vi "Update LCD.vi"(8 "error in":errorcluster, 11 "Data Cluster":T1) -> (0 "error out":errorcluster, 2 "LCD":string, 3 "Module Data":T1)   [LabVIEW 2026, in "Front Panel Emulator.lvlib"]
uses:
  Front Panel Emulator.lvlib
  Module Data--cluster.ctl
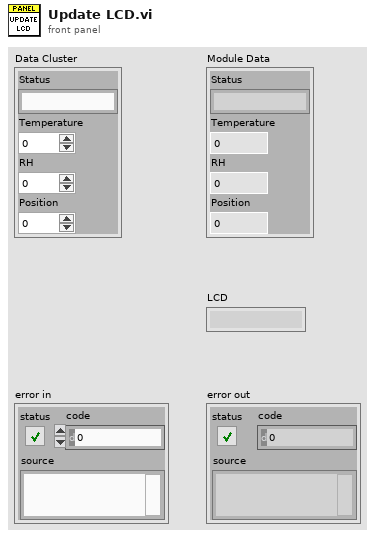
[diagram p1: front panel]
types:
  T1 = typedef "Front Panel Emulator.lvlib/Module Data--cluster.ctl" = cluster{"Status":string, "Temperature":dbl, "RH":dbl, "Position":dbl}
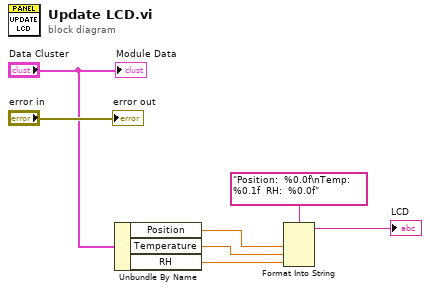
[diagram p0: block diagram]
diagram:
  n1 = Unbundle By Name("Data Cluster") -> ("Position"=w4:dbl, "Temperature"=w5:dbl, "RH"=w6:dbl)
  n2 = Format Into String(format string="Position:  %0.0f\nTemp:  %0.1f  RH:  %0.0f", w4, w5, w6) -> (resulting string=→"LCD":string)  [unwired: 2 in, 1 out]
  "error out" <- "error in"
  "Module Data" <- "Data Cluster"
